vi "Create Sonde Info String Array.vi"(0 "VISA Refnum in":refnum<visa-resource-name>="COM12", 1 "Initialize/Close?":bool=TRUE, 5 "Sensor Address In":string="0", 7 "seconds since 1Jan1904":timestamp, 11 "error in (no error)":errorcluster) -> (4 "VISA Refnum out":refnum<visa-resource-name>, 6 "Address Out":string, 10 "Array":string[][](array[string]), 15 "error out":errorcluster)   [LabVIEW 2016]
panel:
  out "error out 2":errorcluster
  out "read buffer":string
  out "return count":u32
  out "date/time string":string
  out "Serial Number":string
  out "Sensor Version":string
  out "Sensor Model Number":string
  out "Company Name":string
  out "SDI-12 Compatibility Number":dbl
  out "Identification: Address":string
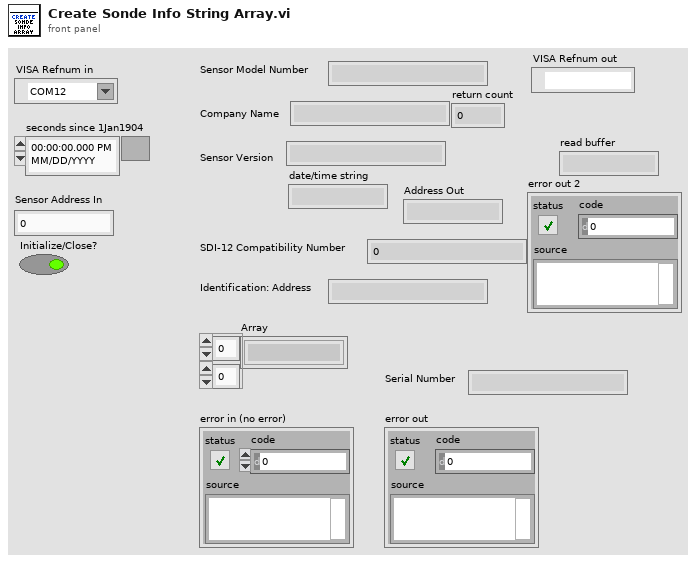
[diagram p1: front panel]
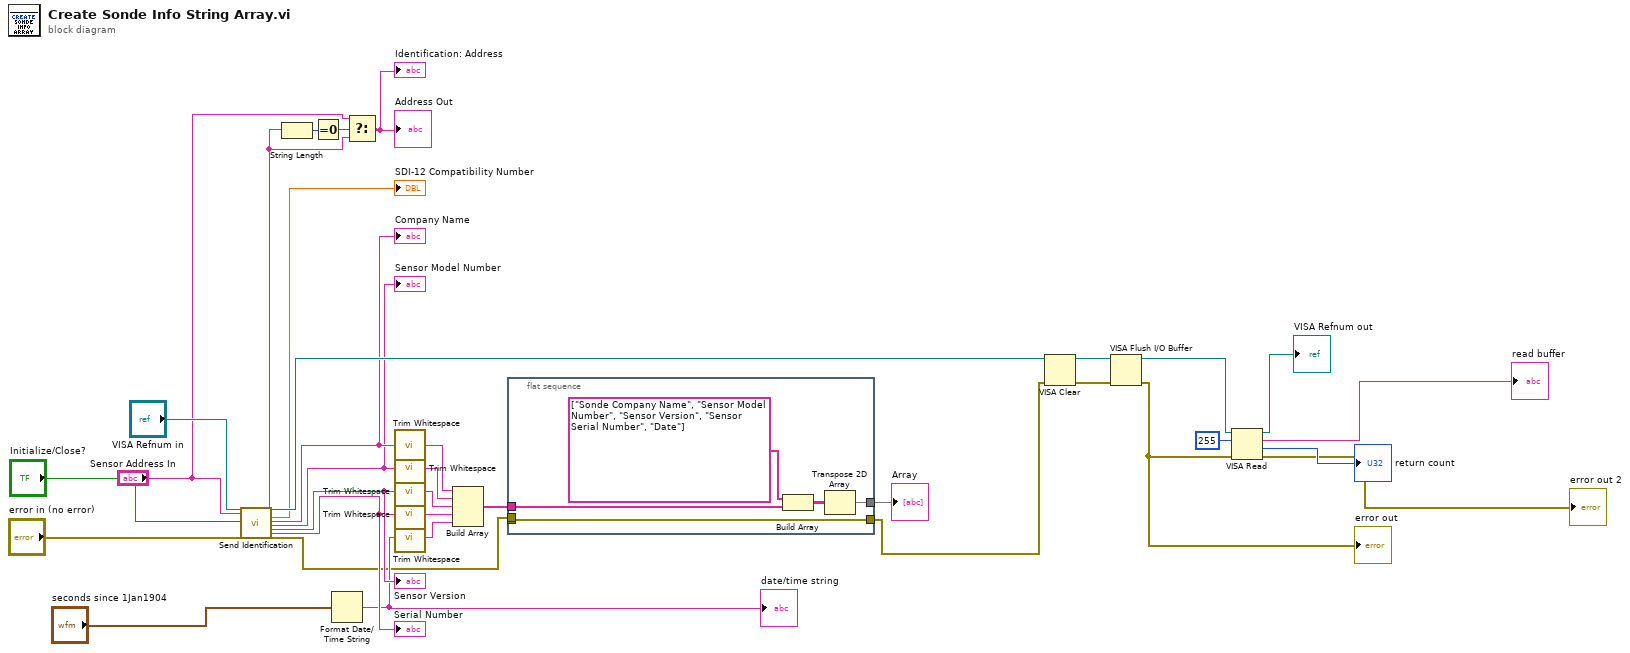
[diagram p0: block diagram]
diagram:
  n1 = call "Send Identification.vi"("RS232 Port In"="VISA Refnum in", "Sensor Address In"="Sensor Address In", "Initialize/Close?"="Initialize/Close?", "Error In (No Error)"="error in (no error)") -> ("RS232 Port Out"=w32:refnum<visa-resource-name>, "Address Out"=w13:string, "SDI-12 Compatibility Number"=→"SDI-12 Compatibility Number":dbl, "Company Name"=w28:string, "Sensor Model Number"=w27:string, "Sensor Version"=w26:string, "Serial Number/MISC"=w25:string, "Error Out"=w17:errorcluster)  [unwired: 16 in]
  "Company Name" <- w28
  "Sensor Model Number" <- w27
  "Sensor Version" <- w26
  "Serial Number" <- w25
  n2 = String Length(string=w13) -> (length=w15:i32)
  n3 = Equal To 0?(x=w15) -> (x = 0?=w14:bool)
  n4 = Format Date/Time String(seconds (now)="seconds since 1Jan1904") -> (date/time string=w23:string)  [unwired: 2 in]
  "date/time string" <- w23
  n5 = Select(t="Sensor Address In", s=w14, f=w13) -> (s? t:f=→"Address Out" →"Identification: Address":string)
  n6 = call <vilib>:"Trim Whitespace.vi"("string"=w28) -> ("trimmed string"=w22:string)  [unwired: 1 in]
  n7 = call <vilib>:"Trim Whitespace.vi"("string"=w27) -> ("trimmed string"=w21:string)  [unwired: 1 in]
  n8 = call <vilib>:"Trim Whitespace.vi"("string"=w26) -> ("trimmed string"=w20:string)  [unwired: 1 in]
  n9 = call <vilib>:"Trim Whitespace.vi"("string"=w25) -> ("trimmed string"=w19:string)  [unwired: 1 in]
  n10 = call <vilib>:"Trim Whitespace.vi"("string"=w23) -> ("trimmed string"=w18:string)  [unwired: 1 in]
  n11 = Build Array(w22, w21, w20, w19, w18) -> (w24:string[])
  n12 = flat-sequence {
    tunnel: w24 -> [w39]
    tunnel: [w36] -> w34
    tunnel: [w35] -> _
    tunnel: w17 -> [w35]
    tunnel: [w35] -> w9
    frame #0 {
      n13 = Build Array(string[] ["Sonde Company Name", "Sensor Model Number", "Sensor Version", "Sensor Serial Number", "Date"] ("appended array 3"), w39) -> (w38:string[][])
      n14 = Transpose 2D Array(2D array=w38) -> (transposed array=w36:string[][])
    }
  }
  n15 = VISA Clear(VISA resource name=w32, error in (no error)=w9) -> (VISA resource name out=w10:refnum<visa-resource-name>, error out=w8:errorcluster)
  n16 = VISA Flush I/O Buffer(VISA resource name=w10, error in (no error)=w8) -> (VISA resource name out=w5:refnum<visa-resource-name>, error out=w6:errorcluster)  [unwired: 1 in]
  "error out" <- w6
  n17 = VISA Read(VISA resource name=w5, byte count=u32 255, error in (no error)=w6) -> (VISA resource name out=→"VISA Refnum out":refnum<visa-resource-name>, read buffer=→"read buffer":string, return count=→"return count":u32, error out=→"error out 2":errorcluster)
  "Array" <- w34
